vi "Create Unique ID.vi"() -> (0 "ID String":string)   [LabVIEW 2014]
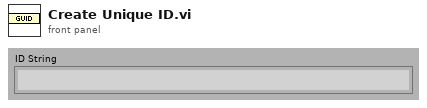
[diagram p1: front panel]
types:
  T1 = cluster{"[0]":u8, "[1]":u8, "[2]":u8, "[3]":u8, "[4]":u8, "[5]":u8, "[6]":u8, "[7]":u8, "[8]":u8, "[9]":u8, "[10]":u8, "[11]":u8, "[12]":u8, "[13]":u8, "[14]":u8, "[15]":u8}
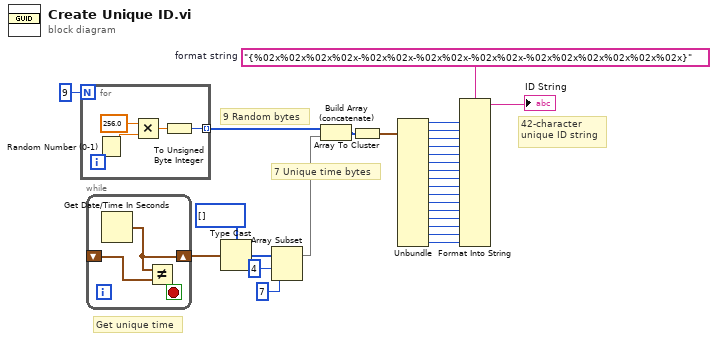
[diagram p0: block diagram]
diagram:
  w2 = "{%02x%02x%02x%02x-%02x%02x-%02x%02x-%02x%02x-%02x%02x%02x%02x%02x%02x}"  # format string
  # "42-character\nunique ID string"
  # "7 Unique time bytes"
  # "9 Random bytes"
  # "Get unique time"
  n1 = for {
    N: 9 -> [_]
    tunnel: [w29] -> w11 mode=indexing
    n2 = Random Number (0-1)() -> (number: 0 to 1=w32:dbl)
    n3 = Multiply(x=256.0, y=w32) -> (x*y=w30:dbl)
    n4 = To Unsigned Byte Integer(number=w30) -> (unsigned 8bit integer=w29:u8)
  }
  n5 = while {
    shift-right: [w35] -> w3
    shift-left: _ -> [w34]
    stop <- w33 stop-if-true
    n6 = Get Date/Time In Seconds() -> (seconds since 1Jan1904=w35:timestamp)
    n7 = Not Equal?(x=w35, y=w34) -> (x != y?=w33:bool)
  }
  n8 = Type Cast(type=u8[] [], x=w3) -> (*(type *) &x=w5:u8[])
  n9 = Array Subset(array=w5, index=4, length=7 ("index")) -> (w8:u8[])
  n10 = Build Array (concatenate)(w11, w8) -> (w9:u8[])
  n11 = Array To Cluster(array=w9) -> (cluster=w28:T1)
  n12 = Unbundle(w28) -> ("[0]"=w27:u8, "[1]"=w26:u8, "[2]"=w25:u8, "[3]"=w24:u8, "[4]"=w23:u8, "[5]"=w22:u8, "[6]"=w21:u8, "[7]"=w20:u8, "[8]"=w19:u8, "[9]"=w18:u8, "[10]"=w17:u8, "[11]"=w16:u8, "[12]"=w15:u8, "[13]"=w14:u8, "[14]"=w13:u8, "[15]"=w12:u8)
  n13 = Format Into String(format string=w2, w27, w26, w25, w24, w23, w22, w21, w20, w19, w18, w17, w16, w15, w14, w13, w12) -> (resulting string=→"ID String":string)  [unwired: 2 in, 1 out]
